vi "Filtra caratteri non numerici.vi"(11 "string in":string) -> (3 "string":string)   [LabVIEW 2019]
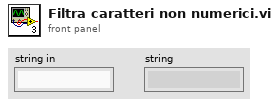
[diagram p1: front panel]
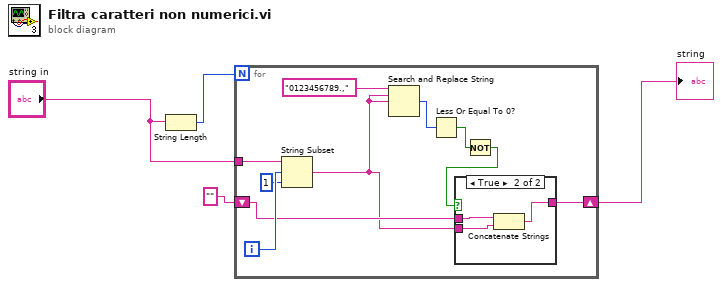
[diagram p0: block diagram]
diagram:
  n1 = String Length(string="string in") -> (length=w2:i32)
  n2 = for {
    N: w2 -> [_]
    tunnel: "string in" -> [w14]
    shift-right: [w5] -> w4
    shift-left: "" ("string") -> [w7]
    i -> [w13]
    n3 = String Subset(string=w14, offset (0)=w13, length (rest)=1 ("length (rest)")) -> (substring=w6:string)
    n4 = Search and Replace String(input string="0123456789.,", search string=w6, replace string=w6) -> (number of replacements=w10:i32)  [unwired: 5 in, 3 out]
    n5 = Less Or Equal To 0?(x=w10) -> (x <= 0?=w9:bool)
    n6 = Not(x=w9) -> (.not. x?=w8:bool)
    n7 = case shown="True" w8 {
      tunnel: w7 -> [w15 w18]
      tunnel: w6 -> [_ w17]
      tunnel: [w15 w16] -> w5
      frame False {
      }
      frame True {
        n8 = Concatenate Strings(w18, w17) -> (w16:string)
      }
    }
  }
  "string" <- w4
